vi "Save Config.vi"(8 "error in (no error)":errorcluster, 11 "picoG in":refnum<class "picoG.lvclass">) -> (0 "error out":errorcluster, 3 "picoG out":refnum<class "picoG.lvclass">)   [LabVIEW 2020, in "PicoG-App.lvlib" / "picoG.lvclass"]
uses:
  picoG.lvclass
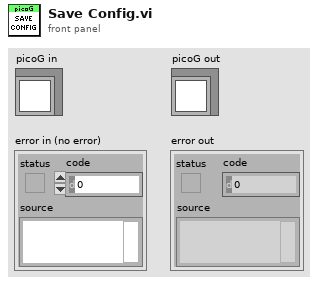
[diagram p1: front panel]
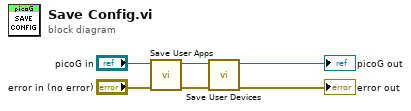
[diagram p0: block diagram]
diagram:
  n1 = call "Save User Apps.vi"("error in (no error)"="error in (no error)", "picoG in"="picoG in") -> ("error out"=w3:errorcluster, "picoG out"=w4:refnum<class "picoG.lvclass">)  [unwired: 8 in]
  n2 = call "Save User Devices.vi"("error in (no error)"=w3, "picoG in"=w4) -> ("error out"=→"error out":errorcluster, "picoG out"=→"picoG out":refnum<class "picoG.lvclass">)  [unwired: 8 in]
